vi "Configure.vi"(7 "Reset":bool, 8 "error in (no error)":errorcluster, 9 "baud rate (9600)":u32=9600, 10 "VISA resource name":refnum<visa-resource-name>="COM6", 11 "Serial Controller in":refnum<class "Serial Controller.lvclass">) -> (0 "error out":errorcluster, 3 "Serial Controller out":refnum<class "Serial Controller.lvclass">)   [LabVIEW 2014, in "Serial Controller.lvclass"]
uses:
  Serial Controller.lvclass
  <vilib>/Instr/_visa.llb/VISA Set IO Buffer Mask.ctl
  Serial Controller.lvclass/Serial Controller.ctl
  <vilib>/Instr/_visa.llb/VISA Configure Serial Port (Instr).vi
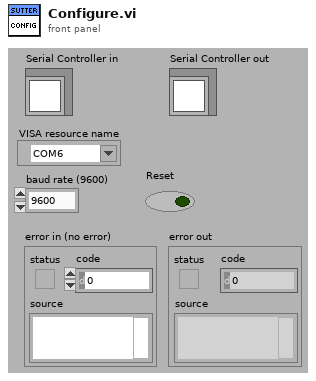
[diagram p1: front panel]
types:
  T1 = typedef "VISA Set IO Buffer Mask.ctl" = u16
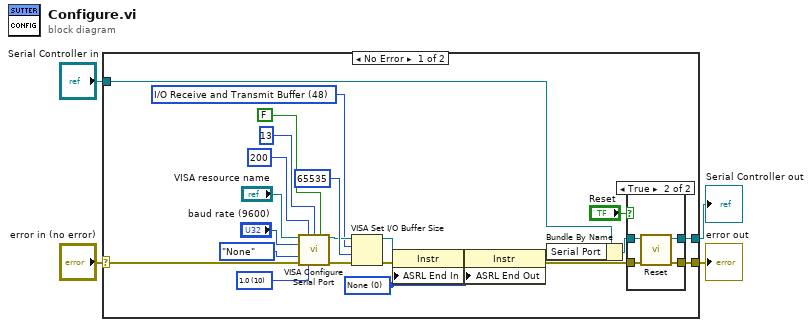
[diagram p0: block diagram]
diagram:
  n1 = case shown="No Error" "error in (no error)" {
    selector: "error in (no error)" -> [w23 w36]
    tunnel: [w15 w36] -> w3
    tunnel: [w16 w35] -> w1
    tunnel: "Serial Controller in" -> [w22 w35]
    frame No Error {
      w12 = u16 0 items=["None", "Last Bit", "TermChar"] ("Serial Settings:End Mode for Reads")
      w14 = T1 48 items=["I/O Receive Buffer"=16, "I/O Transmit Buffer"=32, "I/O Receive and Transmit Buffer"=48] ("Mask")
      w5 = u16 10 items=["1.0"=10, "1.5"=15, "2.0"=20] ("stop bits (10: 1 bit)")
      n2 = call-poly "VISA Configure Serial Port"("VISA resource name"="VISA resource name", "timeout (10sec)"=u32 200, "termination char\n(0xA = '\\n' = LF)"=u8 13 ("termination char\n(0xA = '\\n' = LF)"), "Enable Termination\nChar (T)"=FALSE ("Enable Termination\nChar (T)"), "baud rate (9600)"="baud rate (9600)", "parity (0:none)"=enum16{"None", "Odd", "Even", "Mark", "Space"}."None", "error in (no error)"=w23, "stop bits (10: 1 bit)"=w5) -> ("VISA resource name out"=w20:refnum<visa-resource-name>, "error out"=w19:errorcluster)  [unwired: 6 in]
      n3 = VISA Set I/O Buffer Size(VISA resource name=w20, mask (16)=w14, size (4096)=u32 65535, error in (no error)=w19) -> (VISA resource name out=w10:refnum<visa-resource-name>, error out=w7:errorcluster)
      n4 = property class="Instr"(reference=w10, error in=w7, "ASRL End In"=w12) -> (reference out=w8:refnum<visa-resource-name>, error out=w11:errorcluster)
      n5 = property class="Instr"(reference=w8, error in=w11, "ASRL End Out"=w12) -> (reference out=w9:refnum<visa-resource-name>, error out=w6:errorcluster)
      n6 = Bundle By Name(cluster=w22, "Serial Port"=w9) -> (w17:refnum<class "Serial Controller.lvclass">)
      n7 = case shown="True" "Reset" {
        tunnel: w17 -> [w30 w34]
        tunnel: [w30 w33] -> w16
        tunnel: [w29 w32] -> w15
        tunnel: w6 -> [w29 w31]
        frame False {
        }
        frame True {
          n8 = call-dynamic "Reset.vi"("error in (no error)"=w31, "Serial Controller in"=w34) -> ("error out"=w32:errorcluster, "Serial Controller out"=w33:refnum<class "Serial Controller.lvclass">)  [unwired: 8 in]
        }
      }
    }
    frame Error {
    }
  }
  "error out" <- w3
  "Serial Controller out" <- w1
